vi "WPI_MotorControlScaleToPWM.vi"(10 "Output (1,-1)":dbl, 11 "DeadBand Info":T1={"Name"="", "maxPositivePwm"=0, "minPositivePwm"=0, "centerPwm"=0, "maxNegativePwm"=0, "minNegativePwm"=0, "angularRange"=170}) -> (2 "Raw PWM Value":u16)   [LabVIEW 2025]
doc: "This software is licensed. Open the labview\\readme\\WPI Robotics Library Open Source License.txt file for more information."
uses:
  <vilib>/Rock Robotics/WPI/PWM/WPI_PWMDeadband.ctl
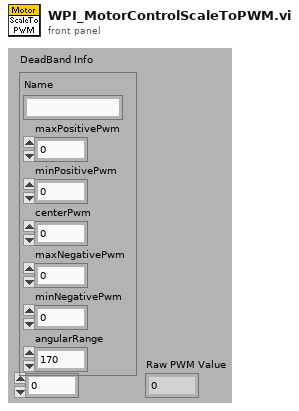
[diagram p1: front panel]
types:
  T1 = typedef "WPI_PWMDeadband.ctl" = cluster{"Name":string, "maxPositivePwm":i32, "minPositivePwm":i32, "centerPwm":i32, "maxNegativePwm":i32, "minNegativePwm":i32, "angularRange":u16}
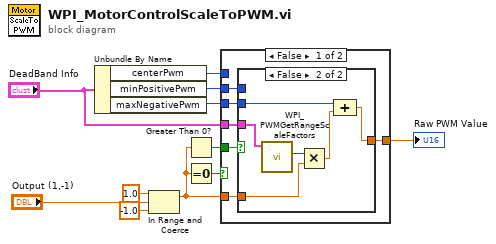
[diagram p0: block diagram]
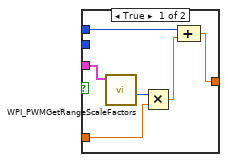
[diagram p2: hidden frame]
diagram:
  n1 = Unbundle By Name("DeadBand Info") -> ("centerPwm"=w9:i32, "minPositivePwm"=w10:i32, "maxNegativePwm"=w11:i32)
  n2 = In Range and Coerce(upper limit=1.0, x="Output (1,-1)", lower limit=-1.0) -> (coerced(x)=w4:dbl)  [unwired: 1 out]
  n3 = Greater Than 0?(x=w4) -> (x > 0?=w5:bool)
  n4 = Equal To 0?(x=w4) -> (x = 0?=w6:bool)
  n5 = case shown="False" w6 {
    tunnel: w5 -> [w17 _]
    tunnel: w4 -> [w16 _]
    tunnel: "DeadBand Info" -> [w15 _]
    tunnel: w10 -> [w14 _]
    tunnel: w11 -> [w13 _]
    tunnel: [w12 w30] -> w1
    tunnel: w9 -> [_ w30]
    frame False {
      n6 = case shown="False" w17 {
        tunnel: w16 -> [w23 w29]
        tunnel: w15 -> [w19 w24]
        tunnel: w14 -> [w21 _]
        tunnel: w13 -> [_ w26]
        tunnel: [w20 w27] -> w12
        frame True {
          n7 = call <vilib>:"WPI_PWMGetRangeScaleFactors.vi"("DeadBand"=w19) -> ("positiveScaleFactor"=w18:i32)  [unwired: 10 out]
          n8 = Multiply(x=w18, y=w23) -> (x*y=w22:dbl)
          n9 = Compound Arithmetic op=ADD(w21, w22) -> (w20:dbl)
        }
        frame False {
          n10 = call <vilib>:"WPI_PWMGetRangeScaleFactors.vi"("DeadBand"=w24) -> ("negativeScaleFactor"=w25:i32)  [unwired: 10 out]
          n11 = Multiply(x=w25, y=w29) -> (x*y=w28:dbl)
          n12 = Compound Arithmetic op=ADD(w26, w28) -> (w27:dbl)
        }
      }
    }
    frame True {
    }
  }
  "Raw PWM Value" <- w1
